vi "SecondLevelThreat_Init.vi"(0 "object in":refnum<class "SecondLevelThreat.lvclass">, 5 "error in (no error)":errorcluster) -> (14 "object out":refnum<class "SecondLevelThreat.lvclass">, 19 "error out":errorcluster)   [LabVIEW 2023, in "SecondLevelThreat.lvclass"]
uses:
  SecondLevelThreat.lvclass
  C:/Users/ebert/Documents/codes/SSL/repo/SSL_AI/NewSTP/Evaluators/Evaluator_class/Evaluator.lvclass
  Criteria/OpenAngleToGoal_class/OpenAngleToGoal.lvclass
  Criteria/PassInterception_class/PassInterception.lvclass
  Criteria/ReceptionAngle_class/ReceptionAngle.lvclass
  C:/Users/ebert/Documents/codes/SSL/repo/SSL_AI/NewSTP/Criteria/Criterion_class/Criterion.lvclass
  Evaluator_class/Evaluator.lvclass
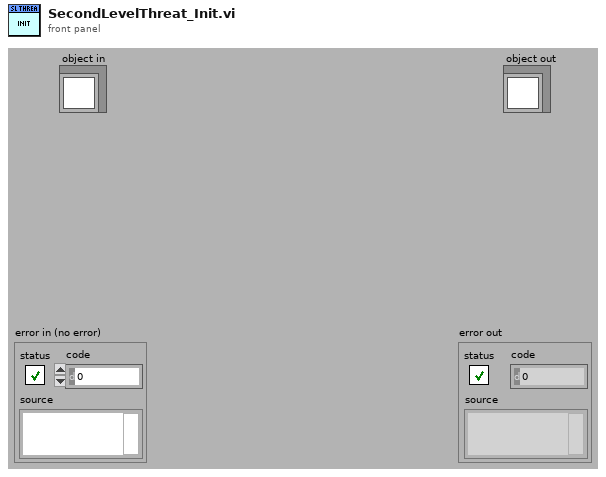
[diagram p1: front panel]
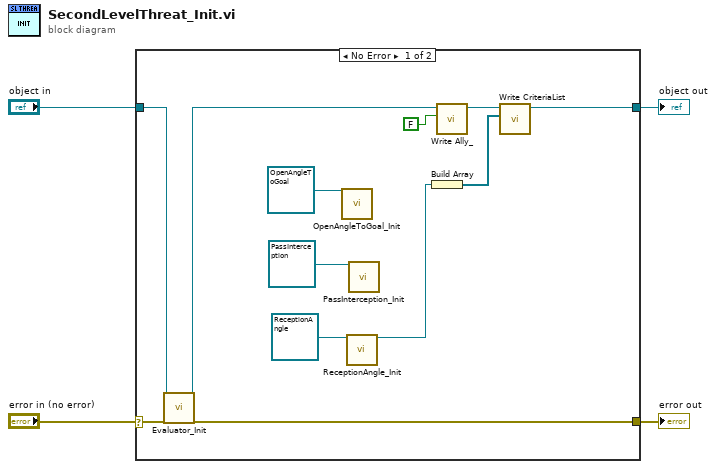
[diagram p0: block diagram]
diagram:
  n1 = case shown="No Error" "error in (no error)" {
    selector: "error in (no error)" -> [w16 w17]
    tunnel: [w11 w18] -> w4
    tunnel: "object in" -> [w14 w18]
    tunnel: [w15 w17] -> w1
    frame No Error {
      n2 = call "Evaluator_Init.vi"("object in"=w14, "error in (no error)"=w16) -> ("object out"=w13:refnum<class "SecondLevelThreat.lvclass">, "error out"=w15:errorcluster)  [unwired: 16 in]
      n3 = call "OpenAngleToGoal_Init.vi"("object in"=refnum<class "OpenAngleToGoal.lvclass"> refnum ("OpenAngleToGoal")) -> ()  [unwired: 17 in, 2 out]
      n4 = call "ReceptionAngle_Init.vi"("object in"=refnum<class "ReceptionAngle.lvclass"> refnum ("ReceptionAngle")) -> ("object out"=w5:refnum<class "ReceptionAngle.lvclass">)  [unwired: 17 in, 1 out]
      n5 = call "PassInterception_Init.vi"("object in"=refnum<class "PassInterception.lvclass"> refnum ("BallInterception")) -> ()  [unwired: 17 in, 2 out]
      n6 = Build Array(w5) -> (w6:refnum<class "ReceptionAngle.lvclass">[])
      n7 = call-dynamic "Write Ally_.vi"("Ally?"=FALSE, "Evaluator in"=w13) -> ("Evaluator out"=w12:refnum<class "SecondLevelThreat.lvclass">)  [unwired: 8 in, 1 out]
      n8 = call-dynamic "Write CriteriaList.vi"("CriteriaList"=w6, "Evaluator in"=w12) -> ("Evaluator out"=w11:refnum<class "SecondLevelThreat.lvclass">)  [unwired: 8 in, 1 out]
    }
    frame Error {
    }
  }
  "object out" <- w4
  "error out" <- w1
